vi "Commit To Database.vi"(8 "error in (no error)":errorcluster, 11 "ExcuseNote in":refnum<class "ExcuseNote.lvclass">) -> (0 "error out":errorcluster, 2 "CommitSuccess(True)":bool=TRUE, 3 "ExcuseNote out":refnum<class "ExcuseNote.lvclass">)   [LabVIEW 2015, in "ExcuseNote.lvclass"]
uses:
  ExcuseNote.lvclass
  <vilib>/addons/database/Auxilliary.llb/DB Tools Column Info.ctl
  <vilib>/addons/database/Auxilliary.llb/DB Tools DataTypes.ctl
  ExcuseNote.lvclass/ExcuseNote.ctl
  g_TypeDefinitions/g_Excuse_Column_Titles.vi
  API/_Database/Database.lvclass
  <vilib>/addons/database/NI_Database_API.lvlib
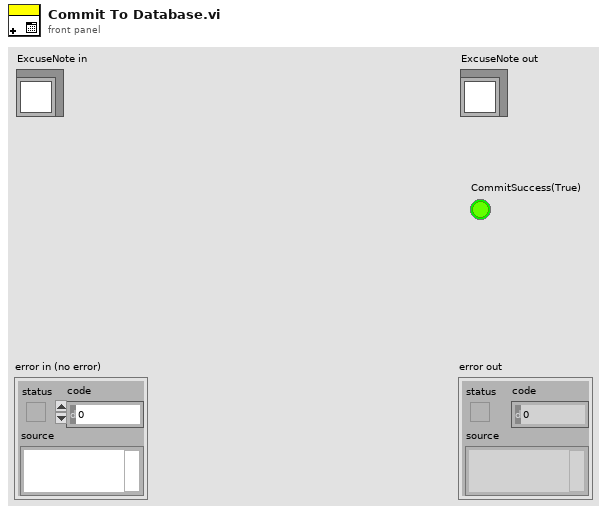
[diagram p1: front panel]
types:
  T1 = typedef "NI_Database_API.lvlib/DB Tools Column Info.ctl" = cluster{"column name":string, "data type":T2, "size":i32, "allow null?":bool}
  T2 = typedef "NI_Database_API.lvlib/DB Tools DataTypes.ctl" = enum16{"String", "Long (I32)", "Single (SGL)", "Double (DBL)", "Date/Time", "Binary"}
  T3 = cluster{"Name(\"\")":string, "ID(\"\")":string, "CurWeek(0)":i32, "请假日期":string, "起始节次":i32, "终止节次":i32, "请假理由":string}
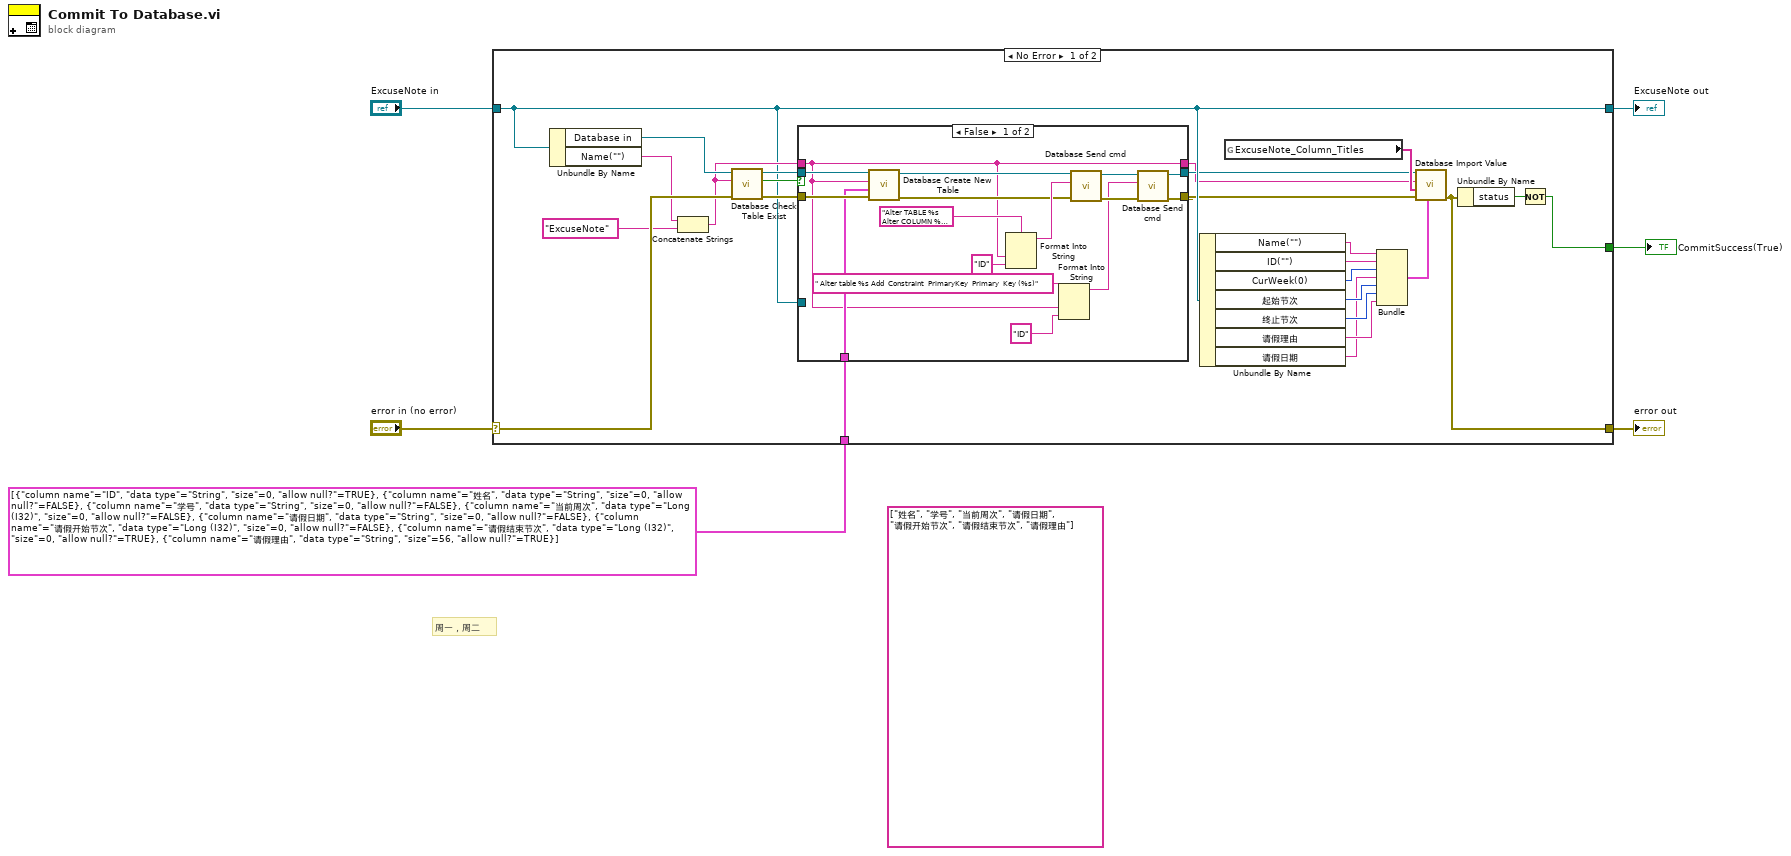
[diagram p0: block diagram]
diagram:
  (unwired) string[] ["姓名", "学号", "当前周次", "请假日期", "请假开始节次", "请假结束节次", "请假理由"] ("ExcuseNote_Column_Titles")
  # "周一，周二"
  n1 = case shown="No Error" "error in (no error)" {
    selector: "error in (no error)" -> [w30 w52]
    tunnel: [w9 w52] -> w5
    tunnel: [w13 w51] -> w3
    tunnel: "ExcuseNote in" -> [w13 w51]
    tunnel: [w10 _] -> w2
    tunnel: T1[] [{"column name"="ID", "data type"=enum."String", "size"=0, "allow null?"=TRUE}, {"column name"="姓名", "data type"=enum."String", "size"=0, "allow null?"=FALSE}, {"column name"="学号", "data type"=enum."String", "size"=0, "allow null?"=FALSE}, {"column name"="当前周次", "data type"=enum."Long (I32)", "size"=0, "allow null?"=FALSE}, {"column name"="请假日期", "data type"=enum."String", "size"=0, "allow null?"=FALSE}, {"column name"="请假开始节次", "data type"=enum."Long (I32)", "size"=0, "allow null?"=FALSE}, {"column name"="请假结束节次", "data type"=enum."Long (I32)", "size"=0, "allow null?"=TRUE}, {"column name"="请假理由", "data type"=enum."String", "size"=56, "allow null?"=TRUE}] ("column information") -> [w23 _]
    frame No Error {
      n2 = Unbundle By Name(w13) -> ("Database in"=w31:refnum<class "Database.lvclass">, "Name(\"\")"=w29:string)
      n3 = Concatenate Strings(w29, "ExcuseNote" ("string")) -> (w24:string)
      n4 = call "Database Check Table Exist.vi"("error in (no error)"=w30, "Table"=w24, "Database in"=w31) -> ("error out"=w25:errorcluster, "Exit?"=w27:bool, "Database out"=w26:refnum<class "Database.lvclass">)  [unwired: 6 in]
      n5 = case shown="False" w27 {
        tunnel: w26 -> [w47 w49]
        tunnel: w25 -> [w46 w50]
        tunnel: w24 -> [w32 w48]
        tunnel: [w35 w50] -> w11
        tunnel: w13 -> [_ _]
        tunnel: w23 -> [w34 _]
        tunnel: [w33 w49] -> w12
        tunnel: [w32 w48] -> w8
        frame False {
          n6 = call "Database Create New Table.vi"("error in (no error)"=w46, "column information"=w34, "table"=w32, "Database in"=w47) -> ("error out"=w37:errorcluster, "Database out"=w36:refnum<class "Database.lvclass">)  [unwired: 6 in]
          n7 = Format Into String(format string="Alter TABLE %s Alter COLUMN %s COUNTER (1, 1)" ("SQL query"), w32, "ID" ("input 2")) -> (resulting string=w45:string)  [unwired: 2 in, 1 out]
          n8 = Format Into String(format string=" Alter table %s Add  Constraint  PrimaryKey  Primary  Key (%s)" ("SQL query"), w32, "ID" ("input 2")) -> (resulting string=w40:string)  [unwired: 2 in, 1 out]
          n9 = call "Database Send cmd.vi"("error in (no error)"=w37, "SQL query"=w45, "Database in"=w36) -> ("error out"=w42:errorcluster, "Database out"=w41:refnum<class "Database.lvclass">)  [unwired: 7 in]
          n10 = call "Database Send cmd.vi"("error in (no error)"=w42, "SQL query"=w40, "Database in"=w41) -> ("error out"=w35:errorcluster, "Database out"=w33:refnum<class "Database.lvclass">)  [unwired: 7 in]
        }
        frame True {
        }
      }
      n11 = Unbundle By Name(w13) -> ("Name(\"\")"=w21:string, "ID(\"\")"=w20:string, "CurWeek(0)"=w15:i32, "起始节次"=w19:i32, "终止节次"=w18:i32, "请假理由"=w17:string, "请假日期"=w7:string)
      n12 = global read "g_Excuse_Column_Titles.vi" "ExcuseNote_Column_Titles"() -> (w22:string[])
      n13 = Bundle("Name(\"\")"=w21, "ID(\"\")"=w20, "CurWeek(0)"=w15, "请假日期"=w7, "起始节次"=w19, "终止节次"=w18, "请假理由"=w17) -> (w16:T3)  [unwired: 1 in]
      n14 = call "Database Import Value.vi"("data"=w16, "error in (no error)"=w11, "columns"=w22, "table"=w8, "object in"=w12) -> ("error out"=w9:errorcluster)  [unwired: 5 in, 1 out]
      n15 = Unbundle By Name(w9) -> ("status"=w14:bool)
      n16 = Not(x=w14) -> (.not. x?=w10:bool)
    }
    frame Error {
    }
  }
  "error out" <- w5
  "ExcuseNote out" <- w3
  "CommitSuccess(True)" <- w2
